vi "Temperature analog value to degrees (SubVI).vi"(11 "Temperature Analog Value":u8) -> (3 "Temperature (C)":dbl)   [LabVIEW 2024]
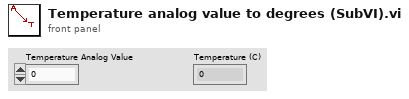
[diagram p1: front panel]
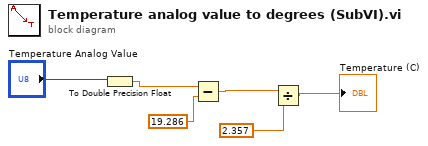
[diagram p0: block diagram]
diagram:
  n1 = To Double Precision Float(number="Temperature Analog Value") -> (double precision float=w2:dbl)
  n2 = Subtract(x=w2, y=19.286) -> (x-y=w4:dbl)
  n3 = Divide(x=w4, y=2.357) -> (x/y=→"Temperature (C)":dbl)
